vi "_Build Create.vi"(8 "error in (no error)":errorcluster, 9 "tableName":string, 10 "DynamicParameters in":refnum<class "DynamicParameters.lvclass">, 11 "SQLConnection in":refnum<class "DBC.lvclass">) -> (0 "error out":errorcluster, 1 "LastIdentityQuery":string, 2 "InsertStatement":string, 3 "SQLConnection out":refnum<class "DBC.lvclass">)   [LabVIEW 2020, in "ORM_DBC_Odbc.lvlib" / "DBC.lvclass"]
uses:
  DBC.lvclass
  C:/Program Files/National Instruments/LabVIEW 2020/vi.lib/Viviota/shared/ORM.lvlibp/ORM/DbConnection/DbConnection.lvclass
  <vilib>/Viviota/shared/ORM.lvlibp/ORM/DynamicParameters/DynamicParameters.lvclass
  <vilib>/Viviota/shared/ORM.lvlibp/ORM/DbConnection/Read LastIdentityQuery.vi
  <vilib>/Viviota/shared/ORM.lvlibp/ORM/DbConnection/Read ColumnNameFormat.vi
  <vilib>/Viviota/shared/ORM.lvlibp/ORM/DynamicParameters/Read ParameterNames.vi
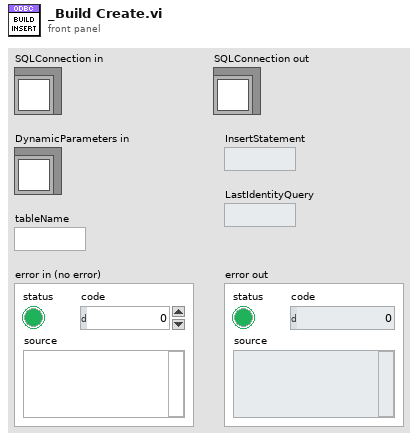
[diagram p1: front panel]
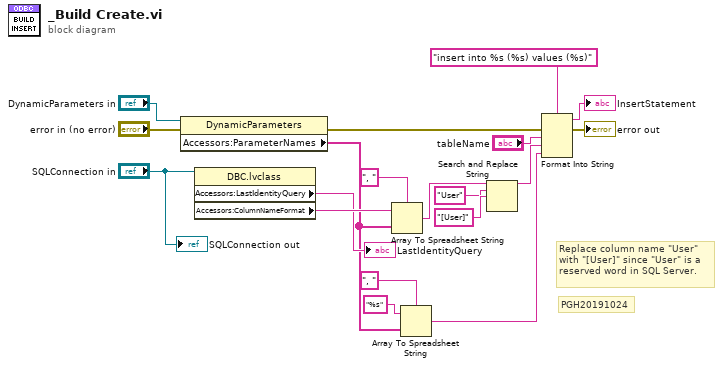
[diagram p0: block diagram]
diagram:
  # "PGH20191024"
  # "Replace column name \"User\"\nwith \"[User]\" since \"User\" is a\nreserved word in SQL Server."
  n1 = property class="DynamicParameters"(reference="DynamicParameters in", error in="error in (no error)") -> (error out=w9:errorcluster, "Accessors:ParameterNames"=w4:string[])  [unwired: 1 out]
  n2 = property class="DBC.lvclass"(reference="SQLConnection in") -> ("Accessors:LastIdentityQuery"=→"LastIdentityQuery":string, "Accessors:ColumnNameFormat"=w15:string)  [unwired: 1 in, 2 out]
  n3 = Array To Spreadsheet String(delimiter (Tab)=", ", array=w4, 3:w15) -> (spreadsheet string=w16:string)
  n4 = Array To Spreadsheet String(delimiter (Tab)=", ", array=w4, 3:"%s" ("format string")) -> (spreadsheet string=w8:string)
  n5 = Search and Replace String(input string=w16, search string="User", replace string="[User]" ("replace string (\"\")")) -> (result string=w17:string)  [unwired: 5 in, 3 out]
  n6 = Format Into String(format string="insert into %s (%s) values (%s)", error in=w9, "tableName", w17, w8) -> (resulting string=→"InsertStatement":string, error out=→"error out":errorcluster)  [unwired: 1 in]
  "SQLConnection out" <- "SQLConnection in"
